vi "Discriminator Slope.vi"(7 "Read Value? (F)":bool, 8 "error in (no error)":errorcluster, 9 "Discriminator Slope (Fall)":T1=enum."Fall", 10 "Discriminator (A)":T2, 11 "VISA resource name":refnum<visa-resource-name>) -> (0 "error out":errorcluster, 1 "Discriminator Slope":T1, 3 "VISA resource name out":refnum<visa-resource-name>)   [LabVIEW 2013, in "SRS SR400.lvlib"]
doc: "<B>DS i { ,j }</B>\n\nThe DS command sets and reads the discriminator slopes. i = 0,1, or 2 designates discriminator A,B, or T and is required. If j is included, the selected discriminator slope is set to RISE, j=0, or FALL, j=1. If j is absent, the slope of discriminator i is returned."
uses:
  <instrlib>/SRS SR400/SRS SR400.lvlib
  <instrlib>/SRS SR400/Public/Typedefs/Discriminator Slope.ctl
  <instrlib>/SRS SR400/Public/Typedefs/Discriminator.ctl
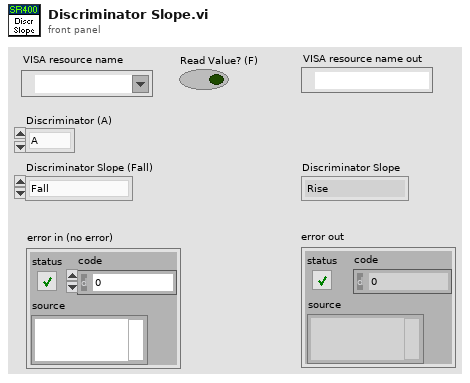
[diagram p1: front panel]
types:
  T1 = typedef "SRS SR400.lvlib/Discriminator Slope.ctl" = enum16{"Rise", "Fall"}
  T2 = typedef "SRS SR400.lvlib/Discriminator.ctl" = enum16{"A", "B", "T"}
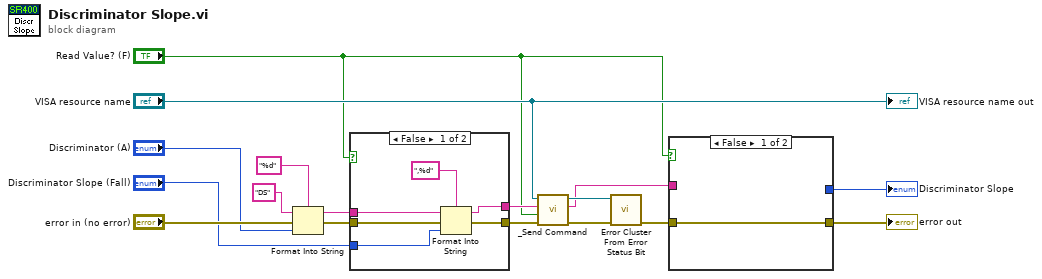
[diagram p0: block diagram]
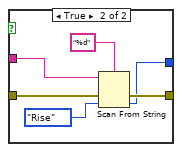
[diagram p2: hidden frame]
diagram:
  n1 = Format Into String(format string="%d", initial string="DS" ("command"), error in="error in (no error)", "Discriminator (A)") -> (resulting string=w15:string, error out=w16:errorcluster)
  n2 = case shown="False" "Read Value? (F)" {
    tunnel: w16 -> [w23 w24]
    tunnel: w15 -> [w18 w25]
    tunnel: [w21 w25] -> w12
    tunnel: [w20 w24] -> w11
    tunnel: "Discriminator Slope (Fall)" -> [w19 _]
    frame False {
      n3 = Format Into String(format string=",%d", initial string=w18, error in=w23, w19) -> (resulting string=w21:string, error out=w20:errorcluster)
    }
    frame True {
    }
  }
  n4 = call <instrlib>:"_Send Command.vi"("error in (no error)"=w11, "Read Value? (F)"="Read Value? (F)", "Command"=w12, "VISA resource name"="VISA resource name") -> ("error out"=w8:errorcluster, "Response"=w5:string, "VISA resource name out"=w9:refnum<visa-resource-name>)  [unwired: 5 out]
  n5 = call <instrlib>:"Error Cluster From Error Status Bit.vi"("error in (no error)"=w8, "VISA resource name"=w9) -> ("error out"=w4:errorcluster)  [unwired: 8 in, 1 out]
  n6 = case shown="False" "Read Value? (F)" {
    tunnel: w5 -> [_ w30]
    tunnel: w4 -> [w26 w32]
    tunnel: [w26 w31] -> w3
    tunnel: [_ w28] -> w2
    frame False {
    }
    frame True {
      n7 = Scan From String(format string="%d", input string=w30, error in=w32, default 1=Discriminator_Slope."Rise" ("Slope")) -> (error out=w31:errorcluster, output 1=w28:T1)  [unwired: 1 in, 2 out]
    }
  }
  "error out" <- w3
  "Discriminator Slope" <- w2
  "VISA resource name out" <- "VISA resource name"
